vi "LED PWM [FPGA].vi"() -> ()   [LabVIEW 2016]
uses:
  <vilib>/Platform/TimedLoop/XDataNode/timing_clust.ctl
  <vilib>/Platform/TimedLoop/XDataNode/nitl_modes.ctl
  <vilib>/Platform/TimedLoop/XDataNode/wakeup.ctl
  <vilib>/rvi/Emulation/niFpgaSctlEmulationGetInTimedLoop.vi
  <vilib>/rvi/Emulation/niFpgaEmulationReportErrorSimple.vi
  <vilib>/rvi/Emulation/niFpgaGetClockAttributes.vi
  <vilib>/rvi/Emulation/niFpgaCriticalErrorInLSC.vi
  <vilib>/rvi/eio/common/nirviEmuTemplateMethod_errors.vi
  <vilib>/Platform/TimedLoop/XDataNode/XDataNode.xnode
  <vilib>/eio/EIONode/EIONode.xnode
  <vilib>/Platform/TimedLoop/XDataNode/XDNodeRunTimeDep.lvlib
panel:
  in  "LED Intensity":u8[](array[numeric])=[0, 0]
  # "LED0"
  # "LED1"
  # "(0 to 255)"
  # "Array of fixed size (2).\nContains green hue\ninformation."
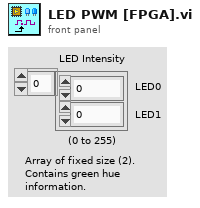
[diagram p1: front panel]
types:
  T1 = typedef "XDNodeRunTimeDep.lvlib/timing_clust.ctl" = cluster{"Expected End [f-1]":u64, "Actual End [f-1]":u64, "Finished Late? [f-1]":bool, "Expected End [i-1]":u64, "Actual End [i-1]":u64, "Finished Late? [i-1]":bool, "Expected Start [i]":u64, "Actual Start [i]":u64, "Expected Start [f]":u64, "Actual Start [f]":u64, "Source Name":string, "Structure Name":string, "Period":i64, "Deadline":i64, "Offset":i64, "Start":i64, "Priority":i32, "Timeout":i32, "Mode":T2, "Wakeup Reason":T3, "Error":errorcluster, "Source Type":string, "Secondary Source Type":string, "Global End Time":u64, "Global Start Time":u64, "Frame Duration":u64, "Iteration Duration":u64, "Assigned CPU":i32, "I/O Scan Engine Mode":u32}
  T2 = typedef "XDNodeRunTimeDep.lvlib/nitl_modes.ctl" = enum32{"No Change", "Process missed periods, maintain original phase", "Discard missed periods, maintain original phase", "Process missed periods, ignore original phase", "Discard missed periods, ignore original phase"}
  T3 = typedef "XDNodeRunTimeDep.lvlib/wakeup.ctl" = enum32{"Normal", "Aborted", "Asynchronous wakeup", "Timing source error", "Timed loop error", "Timeout"}
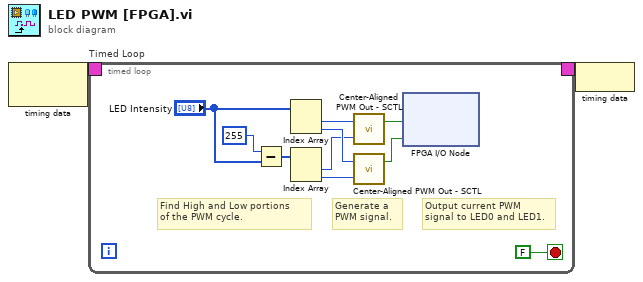
[diagram p0: block diagram]
diagram:
  n1 = node-c288() -> (w2:T1)  [unwired: 1 in]
  n2 = timed-loop "Timed Loop" {
    timing: w2 -> [_]
    timing-out: [_] -> w1
    stop <- FALSE stop-if-true
    # "Output current PWM\nsignal to LED0 and LED1."
    # "Generate a \nPWM signal."
    # "Find High and Low portions \nof the PWM cycle."
    n3 = Subtract(x=u8 255, y="LED Intensity") -> (x-y=w8:u8[])
    n4 = Index Array(array="LED Intensity") -> (element #1=w11:u8, element #2=w7:u8)  [unwired: 2 in]
    n5 = Index Array(array=w8) -> (element #1=w6:u8, element #2=w5:u8)  [unwired: 2 in]
    n6 = call "Center-Aligned PWM Out - SCTL.vi"("Low Pulse"=w6, "High Pulse"=w11) -> ("Output"=w4:bool)  [unwired: 1 in]
    n7 = call "Center-Aligned PWM Out - SCTL.vi"("Low Pulse"=w5, "High Pulse"=w7) -> ("Output"=w3:bool)  [unwired: 1 in]
    n8 = xnode "FPGA I/O Node"("LED0"=w4, "LED1"=w3) -> ()  [unwired: 2 in, 2 out]
  }
  n9 = node-c288(w1) -> ()
